vi "Z Stack Step.vi"(8 "error in (no error)":errorcluster, 10 "Frame Number\n(starts with 1)":i32, 11 "Stage Controller in":refnum<class "Stage Controller.lvclass">) -> (0 "error out":errorcluster, 3 "Stage Controller out":refnum<class "Stage Controller.lvclass">)   [LabVIEW 2023, in "Stage Controller.lvlib" / "Stage Controller.lvclass"]
uses:
  Stage Controller.lvclass
  Stage Controller.lvclass/Stage Controller.ctl
  Stage Axis.ctl
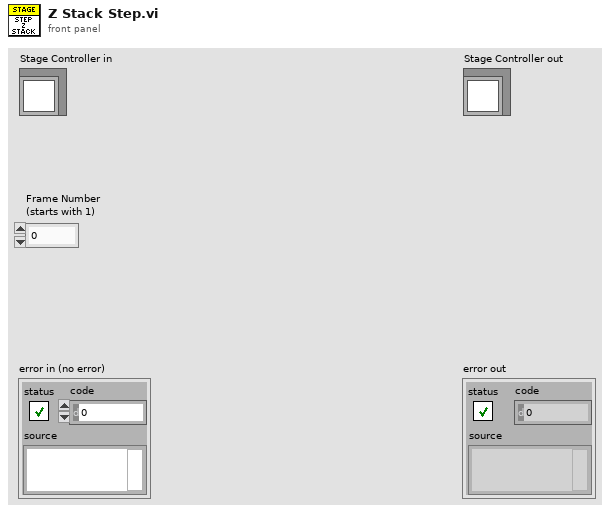
[diagram p1: front panel]
types:
  T1 = typedef "Stage Controller.lvlib/Stage Controller.lvclass/Stage Axis.ctl" = enum16{"unspecified", "X", "Y", "Z"}
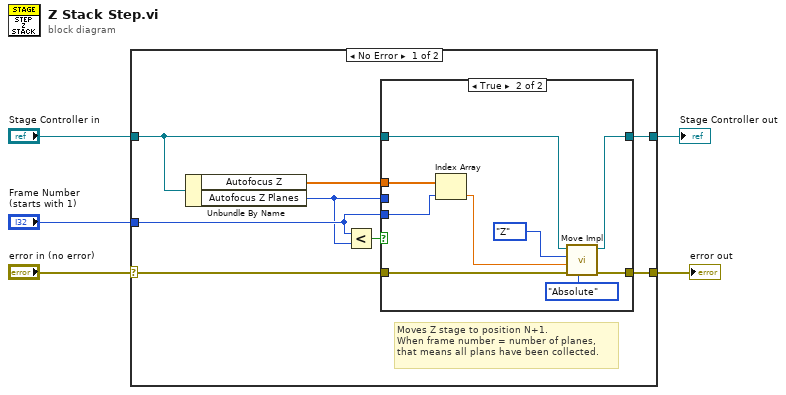
[diagram p0: block diagram]
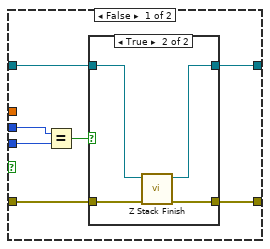
[diagram p2: hidden frame]
diagram:
  n1 = case shown="No Error" "error in (no error)" {
    selector: "error in (no error)" -> [w6 w37]
    tunnel: [w10 w37] -> w4
    tunnel: [w11 w36] -> w1
    tunnel: "Stage Controller in" -> [w7 w36]
    tunnel: "Frame Number\n(starts with 1)" -> [w9 _]
    frame No Error {
      # "Moves Z stage to position N+1.\nWhen frame number = number of planes,\nthat means all plans have been collected."
      n2 = Unbundle By Name(w7) -> ("Autofocus Z"=w13:dbl[], "Autofocus Z Planes"=w8:i32)
      n3 = Less?(x=w9, y=w8) -> (x < y?=w12:bool)
      n4 = case shown="True" w12 {
        tunnel: w7 -> [w16 w31]
        tunnel: [w15 w30] -> w11
        tunnel: w6 -> [w18 w33]
        tunnel: [w17 w32] -> w10
        tunnel: w13 -> [_ w35]
        tunnel: w9 -> [w20 w34]
        tunnel: w8 -> [w19 _]
        frame False {
          n5 = Equal?(x=w19, y=w20) -> (x = y?=w14:bool)
          n6 = case shown="True" w14 {
            tunnel: w18 -> [w21 w26]
            tunnel: [w21 w25] -> w17
            tunnel: w16 -> [w22 w24]
            tunnel: [w22 w23] -> w15
            frame False {
              # "Ignore extra frames\nafter acquisition is\ncomplete (if any)."
            }
            frame True {
              n7 = call-dynamic "Z Stack Finish.vi"("error in (no error)"=w26, "Stage Controller in"=w24) -> ("error out"=w25:errorcluster, "Stage Controller out"=w23:refnum<class "Stage Controller.lvclass">)  [unwired: 8 in]
            }
          }
        }
        frame True {
          n8 = Index Array(array=w35, index=w34) -> (element=w28:dbl)
          n9 = call-dynamic "Move Impl.vi"("Mode"=enum16{"Relative", "Absolute"}."Absolute", "error in (no error)"=w33, "Value (mm)"=w28, "Axis"=Stage_Axis."Z", "Stage Controller in"=w31) -> ("error out"=w32:errorcluster, "Stage Controller out"=w30:refnum<class "Stage Controller.lvclass">)  [unwired: 5 in]
        }
      }
    }
    frame Error {
    }
  }
  "error out" <- w4
  "Stage Controller out" <- w1
